vi "Example calibration data preprocessing.vi"(0 "Vout_cal (V)":dbl[](array[numeric])=[0.091592760722, 1.0386908302, 1.2815961749, 1.472527963, 1.7426600622, 1.8203625132, 2.0411978022, 2.0770638682, 2.2738904915, 2.2840504786, 2.4351853116, 2.4850255178, 2.5605488764], 5 "U_cal (m/s)":dbl[](array[numeric])=[0.29667635602, 1.1301571376, 1.5324625785, 1.9267451591, 2.7016264552, 2.9699742904, 3.8087503579, 3.9703565821, 4.8688444428, 4.9228999336, 5.7326085821, 6.0210422984, 6.4593328997], 7 "Ta_cal (°C)":dbl[](array[numeric])=[20.433095956, 20.435468619, 20.432966163, 20.434483817, 20.437349503, 20.435590331, 20.437475439, 20.43820383, 20.433738789, 20.433883647, 20.444046858, 20.449827253, 20.452159398], 9 "Overheat ratio":dbl=1.7, 11 "Gain":dbl=10.0, 12 "Offset (V)":dbl=0.512) -> (4 "Calibration data":T1={"X cal.[]"=[0.18323830295620053, 0.5022759108677167, 0.5926494582411277, 0.6661572393359195, 0.7738522670991032, 0.8056162976693839, 0.8978854253288069, 0.9131465104685323, 0.998198602505461, 1.0026536354542668, 1.0697031684682123, 1.0921294784978217, 1.12634848007751], "Re cal.[]"=[0.05836901900647489, 0.22234941748039563, 0.3015014894413766, 0.37907259878050203, 0.5315212662031547, 0.5843186336351215, 0.7493379557739939, 0.7811312845686427, 0.9579100635301298, 0.968544779466997, 1.1278235480081842, 1.1845542549316277, 1.2707750850078616], "a1[]"=[0.5139845410306613, 0.694908421100499, 0.9655549133380104, 1.2354182702612118, 1.5388668488196042, 1.7253155968767342, 1.935875310920986, 2.080885331144939, 2.2328002605238204, 2.3813313947618693, 2.452594226248764, 2.5246632991683033], "a2[]"=[-0.567092642319511, 3.0111150428522957, -0.009461861177446703, 2.2004140825264833, 5.776179850523374, -0.22907956125341525, 19.477407826803766, -1.871103511573675, 70.58084557623488, -1.3220160025433672, 7.094218596447346, -0.2914365144530001], "a3[]"=[1.7775103256064757, -11.166529475918521, 16.733581628717324, -4.900141213800908, -59.63298736273686, 9.899216022714324, -643.3109334585097, 21.66651332028892, -8067.401298929666, 18.428518110921583, -163.1245085960374, 4.25840177969994]})   [LabVIEW 2021]
doc: "Example VI for how to pre-process recorded speed & voltage arrays into calibration data using the minimum of inputs.\nPN 16-FEB-24."
uses:
  Ctls/Calibration data.ctl
panel:
  out "Calibration curve":cluster{dbl[], dbl[]}(graph)={[0.18323830295620053, 0.5022759108677167, 0.5926494582411277, 0.6661572393359195, 0.7738522670991032, 0.8056162976693839, 0.8978854253288069, 0.9131465104685323, 0.998198602505461, 1.0026536354542668, 1.0697031684682123, 1.0921294784978217, 1.12634848007751], [0.05836901900647489, 0.22234941748039563, 0.3015014894413766, 0.37907259878050203, 0.5315212662031547, 0.5843186336351215, 0.7493379557739939, 0.7811312845686427, 0.9579100635301298, 0.968544779466997, 1.1278235480081842, 1.1845542549316277, 1.2707750850078616]}
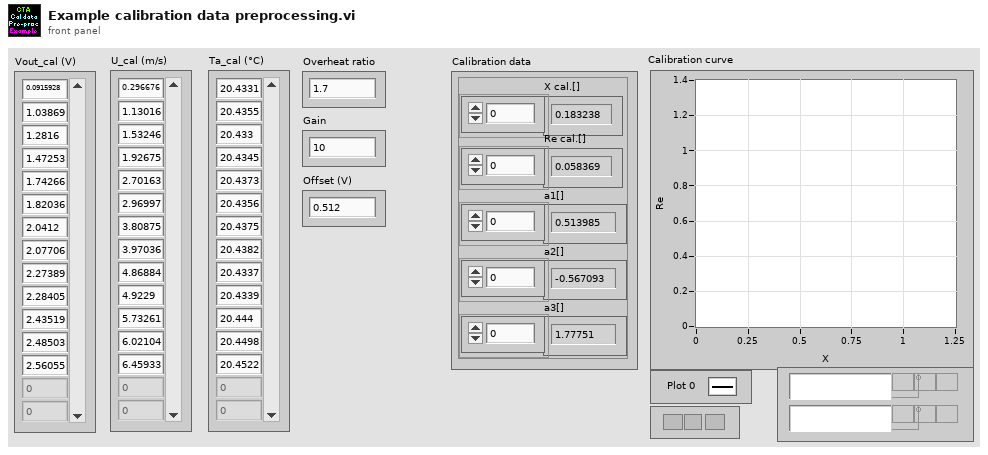
[diagram p1: front panel]
types:
  T1 = typedef "Calibration data.ctl" = cluster{"X cal.[]":dbl[], "Re cal.[]":dbl[], "a1[]":dbl[], "a2[]":dbl[], "a3[]":dbl[]}
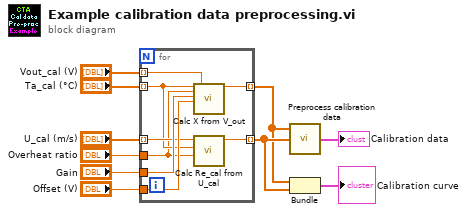
[diagram p0: block diagram]
diagram:
  n1 = for {
    tunnel: [w18] -> w3 mode=indexing
    tunnel: [w17] -> w2 mode=indexing
    tunnel: "Vout_cal (V)" -> [w16] mode=indexing
    tunnel: "Ta_cal (°C)" -> [w12] mode=indexing
    tunnel: "Overheat ratio" -> [w11]
    tunnel: "Gain" -> [w15]
    tunnel: "Offset (V)" -> [w14]
    tunnel: "U_cal (m/s)" -> [w13] mode=indexing
    n2 = call "Calc X from V_out.vi"("Ta (°C)"=w12, "Overheat ratio (Rw / R0)"=w11, "Gain"=w15, "Offset (V)"=w14, "V_out (V)"=w16) -> ("X"=w17:dbl)  [unwired: 14 in]
    n3 = call "Calc Re_cal from U_cal.vi"("Overheat ratio (Rw / R0)"=w11, "Ta (°C)"=w12, "U_cal (m/s)"=w13) -> ("Re"=w18:dbl)  [unwired: 8 in]
  }
  n4 = call "Preprocess calibration data.vi"("Re cal.[]"=w3, "X cal.[]"=w2) -> ("Calibration data"=→"Calibration data":T1)  [unwired: 1 in]
  n5 = Bundle(w2, w3) -> (→"Calibration curve":cluster{dbl[], dbl[]})  [unwired: 1 in]
